vi "Get Joystick.vi"(1 "Operator POVs":i16[](array[numeric]), 2 "Driver Axes":dbl[](array[numeric]), 3 "Operator Buttons":bool[](array[boolean]), 4 "Operator Axes":dbl[](array[numeric]), 5 "Driver POVs":i16[](array[numeric]), 6 "Driver Buttons":bool[](array[boolean])) -> (0 "Joystick Controls Out":T1={"Driver Left Joystick X"=0.0, "Driver Left Joystick Y"=0.0, "Driver A Button"=FALSE, "Driver B Button"=FALSE, "Driver X Button"=FALSE, "Driver Y Button"=FALSE, "Driver Left Bumper"=FALSE, "Driver Right Bumper"=FALSE, "Driver View Button"=FALSE, "Driver Menu Button"=FALSE, "Driver Left Joystick Press"=FALSE, "Driver Right Joystick Press"=FALSE, "Driver Left Trigger"=0.0, "Driver Right Joystick X"=0.0, "Driver Right Joystick Y"=0.0, "Driver Right Trigger"=0.0, "Operator Left Joystick X"=0.0, "Operator Left Joystick Y"=0.0, "Operator A Button"=FALSE, "Operator B Button"=FALSE, "Operator X Button"=FALSE, "Operator Y Button"=FALSE, "Operator Left Bumper"=FALSE, "Operator Right Bumper"=FALSE, "Operator View Button"=FALSE, "Operator Menu Button"=FALSE, "Operator Left Joystick Press"=FALSE, "Operator Right Joystick Press"=FALSE, "Operator Left Trigger"=0.0, "Operator Right Joystick X"=0.0, "Operator Right Joystick Y"=0.0, "Operator Right Trigger"=0.0, "Driver D-Pad"=-1, "Operator D-Pad"=-1})   [LabVIEW 2018]
uses:
  Joystick Controls.ctl
panel:
  in  "Joystick Controls Typedef":T1={"Driver Left Joystick X"=0.0, "Driver Left Joystick Y"=0.0, "Driver A Button"=FALSE, "Driver B Button"=FALSE, "Driver X Button"=FALSE, "Driver Y Button"=FALSE, "Driver Left Bumper"=FALSE, "Driver Right Bumper"=FALSE, "Driver View Button"=FALSE, "Driver Menu Button"=FALSE, "Driver Left Joystick Press"=FALSE, "Driver Right Joystick Press"=FALSE, "Driver Left Trigger"=0.0, "Driver Right Joystick X"=0.0, "Driver Right Joystick Y"=0.0, "Driver Right Trigger"=0.0, "Operator Left Joystick X"=0.0, "Operator Left Joystick Y"=0.0, "Operator A Button"=FALSE, "Operator B Button"=FALSE, "Operator X Button"=FALSE, "Operator Y Button"=FALSE, "Operator Left Bumper"=FALSE, "Operator Right Bumper"=FALSE, "Operator View Button"=FALSE, "Operator Menu Button"=FALSE, "Operator Left Joystick Press"=FALSE, "Operator Right Joystick Press"=FALSE, "Operator Left Trigger"=0.0, "Operator Right Joystick X"=0.0, "Operator Right Joystick Y"=0.0, "Operator Right Trigger"=0.0, "Driver D-Pad"=-1, "Operator D-Pad"=-1}
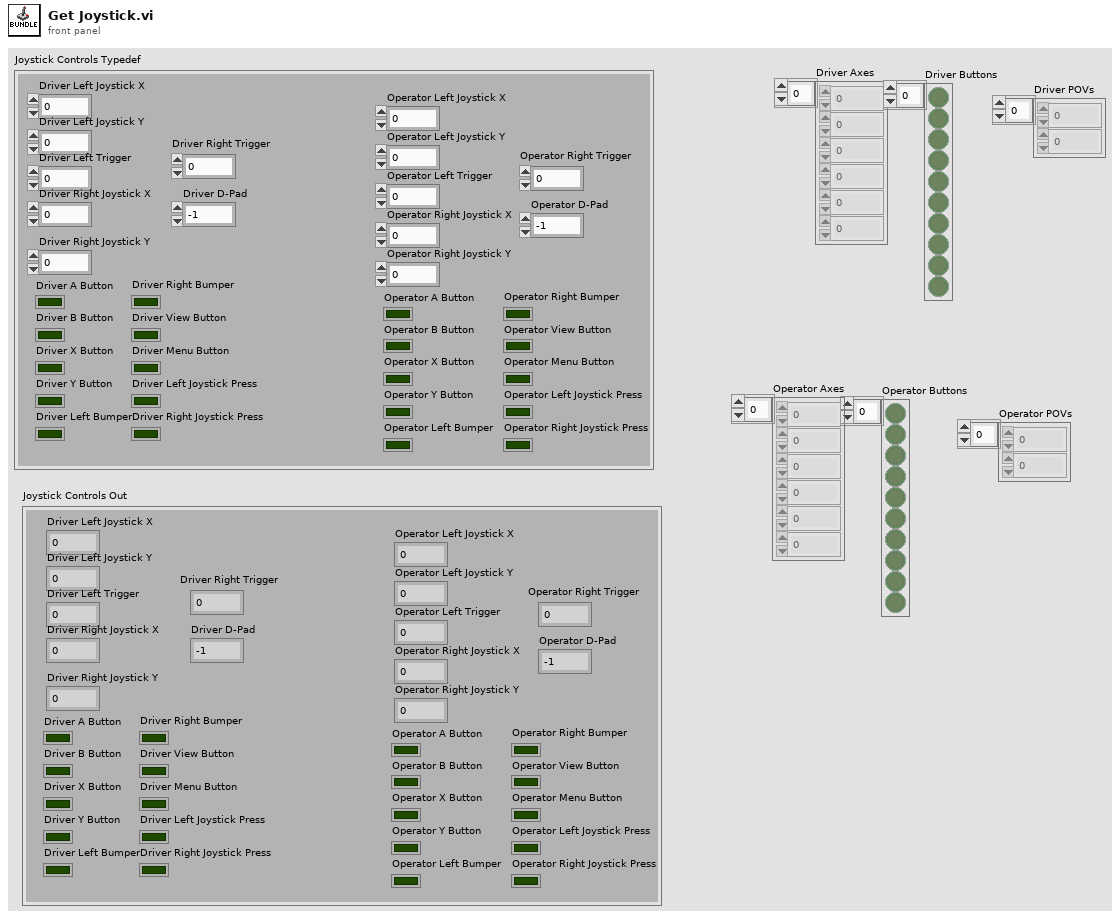
[diagram p1: front panel]
types:
  T1 = typedef "Joystick Controls.ctl" = cluster{"Driver Left Joystick X":dbl, "Driver Left Joystick Y":dbl, "Driver A Button":bool, "Driver B Button":bool, "Driver X Button":bool, "Driver Y Button":bool, "Driver Left Bumper":bool, "Driver Right Bumper":bool, "Driver View Button":bool, "Driver Menu Button":bool, "Driver Left Joystick Press":bool, "Driver Right Joystick Press":bool, "Driver Left Trigger":dbl, "Driver Right Joystick X":dbl, "Driver Right Joystick Y":dbl, "Driver Right Trigger":dbl, "Operator Left Joystick X":dbl, "Operator Left Joystick Y":dbl, "Operator A Button":bool, "Operator B Button":bool, "Operator X Button":bool, "Operator Y Button":bool, "Operator Left Bumper":bool, "Operator Right Bumper":bool, "Operator View Button":bool, "Operator Menu Button":bool, "Operator Left Joystick Press":bool, "Operator Right Joystick Press":bool, "Operator Left Trigger":dbl, "Operator Right Joystick X":dbl, "Operator Right Joystick Y":dbl, "Operator Right Trigger":dbl, "Driver D-Pad":i16, "Operator D-Pad":i16}
  T2 = cluster{"Driver Axes[0]":dbl, "Driver Axes[1]":dbl, "Driver Axes[2]":dbl, "Driver Axes[3]":dbl, "Driver Axes[4]":dbl, "Driver Axes[5]":dbl, "Driver Axes[6]":dbl, "Driver Axes[7]":dbl, "Driver Axes[8]":dbl}
  T3 = cluster{"Operator Axes[0]":dbl, "Operator Axes[1]":dbl, "Operator Axes[2]":dbl, "Operator Axes[3]":dbl, "Operator Axes[4]":dbl, "Operator Axes[5]":dbl, "Operator Axes[6]":dbl, "Operator Axes[7]":dbl, "Operator Axes[8]":dbl}
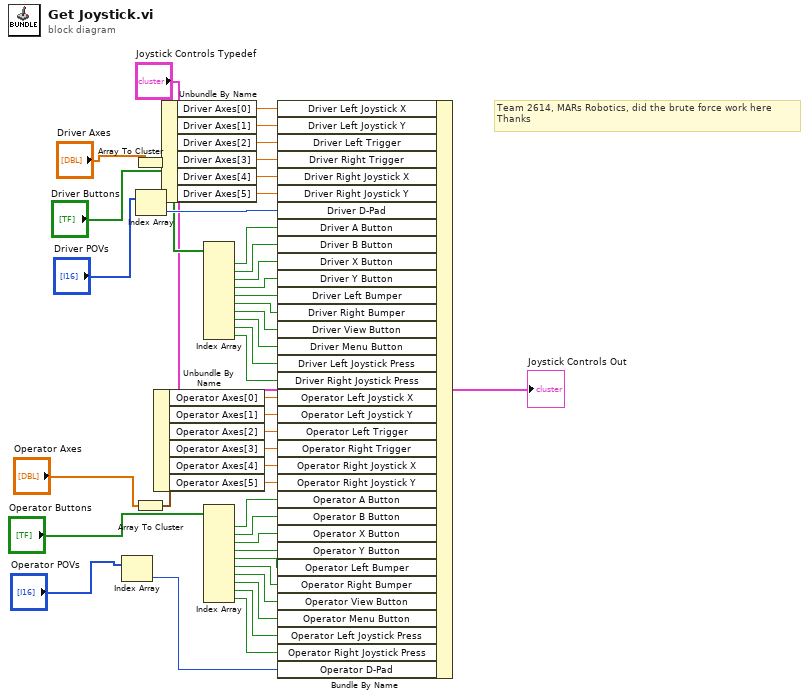
[diagram p0: block diagram]
diagram:
  # "Team 2614, MARs Robotics, did the brute force work here\nThanks"
  n1 = Index Array(array="Operator POVs") -> (element=w9:i16)  [unwired: 1 in]
  n2 = Array To Cluster(array="Driver Axes") -> (cluster=w43:T2)
  n3 = Array To Cluster(array="Operator Axes") -> (cluster=w1:T3)
  n4 = Index Array(array="Driver POVs") -> (element=w10:i16)  [unwired: 1 in]
  n5 = Unbundle By Name(w1) -> ("Operator Axes[0]"=w26:dbl, "Operator Axes[1]"=w25:dbl, "Operator Axes[2]"=w24:dbl, "Operator Axes[3]"=w23:dbl, "Operator Axes[4]"=w22:dbl, "Operator Axes[5]"=w21:dbl)
  n6 = Unbundle By Name(w43) -> ("Driver Axes[0]"=w42:dbl, "Driver Axes[1]"=w41:dbl, "Driver Axes[2]"=w40:dbl, "Driver Axes[3]"=w39:dbl, "Driver Axes[4]"=w38:dbl, "Driver Axes[5]"=w37:dbl)
  n7 = Index Array(array="Driver Buttons") -> (element #1=w36:bool, element #2=w35:bool, element #3=w34:bool, element #4=w33:bool, element #5=w32:bool, element #6=w31:bool, element #7=w30:bool, element #8=w29:bool, element #9=w28:bool, element #10=w27:bool)  [unwired: 10 in]
  n8 = Index Array(array="Operator Buttons") -> (element #1=w20:bool, element #2=w19:bool, element #3=w18:bool, element #4=w17:bool, element #5=w15:bool, element #6=w16:bool, element #7=w14:bool, element #8=w13:bool, element #9=w12:bool, element #10=w11:bool)  [unwired: 10 in]
  n9 = Bundle By Name(cluster="Joystick Controls Typedef", "Driver Left Joystick X"=w42, "Driver Left Joystick Y"=w41, "Driver Left Trigger"=w40, "Driver Right Trigger"=w39, "Driver Right Joystick X"=w38, "Driver Right Joystick Y"=w37, "Driver D-Pad"=w10, "Driver A Button"=w36, "Driver B Button"=w35, "Driver X Button"=w34, "Driver Y Button"=w33, "Driver Left Bumper"=w32, "Driver Right Bumper"=w31, "Driver View Button"=w30, "Driver Menu Button"=w29, "Driver Left Joystick Press"=w28, "Driver Right Joystick Press"=w27, "Operator Left Joystick X"=w26, "Operator Left Joystick Y"=w25, "Operator Left Trigger"=w24, "Operator Right Trigger"=w23, "Operator Right Joystick X"=w22, "Operator Right Joystick Y"=w21, "Operator A Button"=w20, "Operator B Button"=w19, "Operator X Button"=w18, "Operator Y Button"=w17, "Operator Left Bumper"=w15, "Operator Right Bumper"=w16, "Operator View Button"=w14, "Operator Menu Button"=w13, "Operator Left Joystick Press"=w12, "Operator Right Joystick Press"=w11, "Operator D-Pad"=w9) -> ()  [unwired: 1 out]
  "Joystick Controls Out" <- "Joystick Controls Typedef"
